vi "Haupt VI.vi"() -> ()   [LabVIEW 2024]
panel:
  out "Umfang":dbl
  out "Fläche":dbl
  out "error out":errorcluster
  in  "error in (no error)":errorcluster
  in  "stop":bool
  in  "OK Button":bool
  in  "Breite":dbl
  in  "Länge":dbl
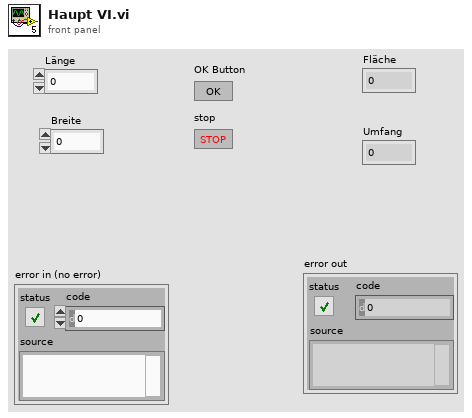
[diagram p1: front panel]
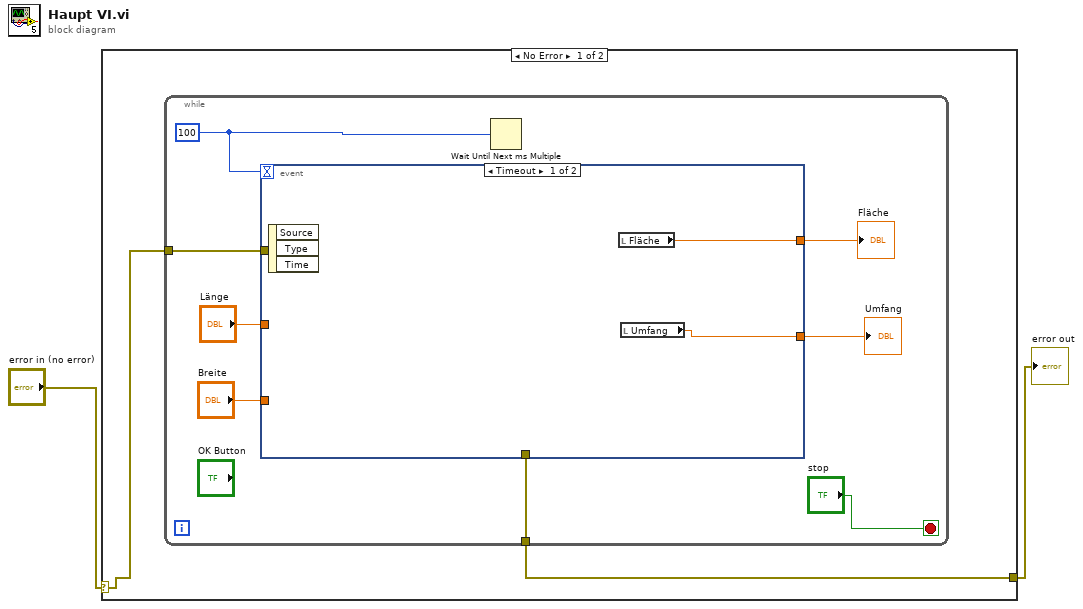
[diagram p0: block diagram]
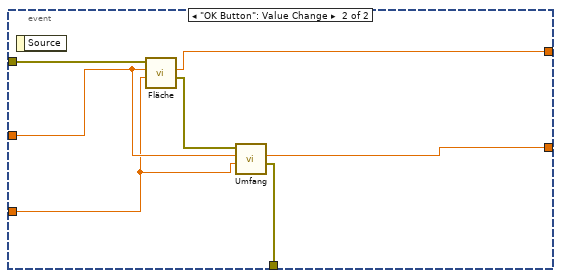
[diagram p2: hidden frame]
diagram:
  n1 = case shown="No Error" "error in (no error)" {
    selector: "error in (no error)" -> [w4 w22]
    tunnel: [w3 w22] -> w1
    frame No Error {
      n2 = while {
        tunnel: w4 -> [w9]
        tunnel: [w5] -> w3
        stop <- "stop" stop-if-true
        w11 = u32 100 ("millisecond multiple")
        n3 = event shown="[0] Timeout" {
          selector: _ -> [_ _]
          dyn-events: _ -> [_ _]
          timeout: w11 -> [_ _]
          tunnel: "Länge" -> [_ w19]
          tunnel: w9 -> [_ w21]
          tunnel: "Breite" -> [_ w18]
          tunnel: [w13 w20] -> w7
          tunnel: [w14 w16] -> w6
          tunnel: [_ w15] -> w5
          event Timeout {
            n4 = event-data() -> ()  [unwired: 1 in, 3 out]
            n5 = local read "Fläche"() -> (w13:dbl)
            n6 = local read "Umfang"() -> (w14:dbl)
          }
          event "OK Button": Value Change {
            n7 = event-data() -> ()  [unwired: 1 in, 1 out]
            n8 = call "Fläche.vi"("Numeric 2"=w18, "Numeric"=w19, "error in (no error)"=w21) -> ("error out"=w17:errorcluster, "Numeric 3"=w20:dbl)  [unwired: 7 in]
            n9 = call "Umfang.vi"("Breite"=w18, "Länge"=w19, "error in (no error)"=w17) -> ("error out"=w15:errorcluster, "Umfang"=w16:dbl)  [unwired: 7 in]
          }
        }
        "Fläche" <- w7
        "Umfang" <- w6
        n10 = Wait Until Next ms Multiple(millisecond multiple=w11) -> ()  [unwired: 1 out]
      }
    }
    frame Error {
    }
  }
  "error out" <- w1
